vi "Teleop.vi"(10 "Match Info":T1={"Autonomous Elapsed Seconds"=0.0, "TeleOp Elapsed Seconds"=0.0, "Disabled Elapsed Seconds"=0.0, "Visited Autonomous"=FALSE, "Visited TeleOp"=FALSE, "Visited Disabled"=FALSE, "Autonomous Settings"={"Autonomous Style"=enum."Independent", "VI Refnum"=refnum}}, 11 "Call Context":T2) -> ()   [LabVIEW 2020]
doc: "This VI is called for each TeleOp packet received from the DS where the robot is not disabled. It is often used to read from the joysticks and update I/O or to update setpoints for timed control loops. It should complete and return within 20 milliseconds or it may miss DS packets."
uses:
  <vilib>/Rock Robotics/WPI/DriverStation/WPI_DriverStationDerivedRobotMode.ctl
  <vilib>/Rock Robotics/WPI/DriverStation/WPI_DriverStationMatch Info.ctl
  <vilib>/Rock Robotics/WPI/Utilities/WPI_GetSetVariantRefNum.vi
  <vilib>/Rock Robotics/Network Tables/NT Write Boolean Array.vi
  <vilib>/Rock Robotics/Network Tables/NT Write Numeric Array.vi
  Subsystems/Climber/climber_globals.vi
  Subsystems/Shooter/shooter_globals.vi
  Subsystems/Magazine/magazine_globals.vi
  Subsystems/Swerve/swerve_globals.vi
  TitanLib/Lib/TitanLib.lvlib
panel:
  out "Loop Time (ms)":u32(graph)
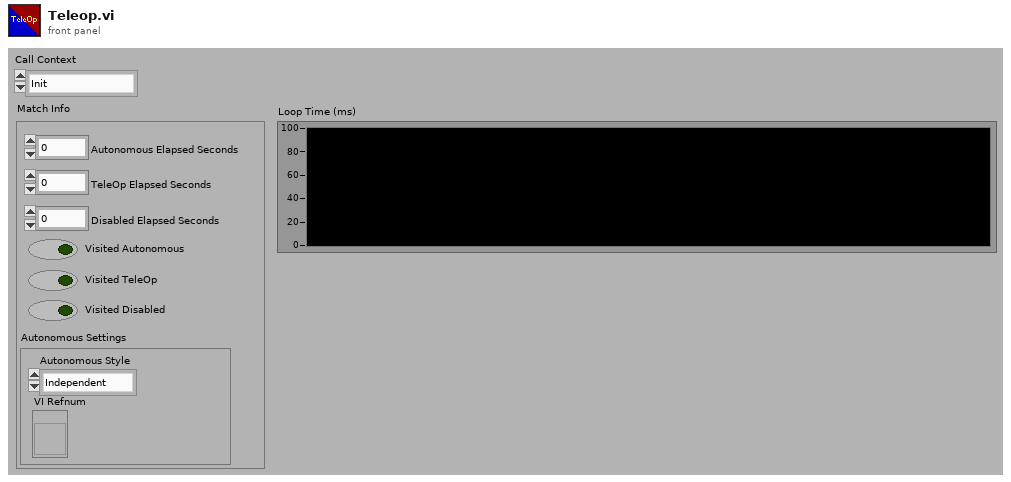
[diagram p1: front panel]
types:
  T1 = typedef "WPI_DriverStationMatch Info.ctl" = cluster{"Autonomous Elapsed Seconds":dbl, "TeleOp Elapsed Seconds":dbl, "Disabled Elapsed Seconds":dbl, "Visited Autonomous":bool, "Visited TeleOp":bool, "Visited Disabled":bool, "Autonomous Settings":cluster{"Autonomous Style":enum16{"Iterative", "Independent"}, "VI Refnum":refnum<vi>}}
  T2 = typedef "WPI_DriverStationDerivedRobotMode.ctl" = enum16{"Init", "Execute", "Stop"}
  T3 = cluster{"Left Stick X":dbl, "Left Stick Y":dbl, "Left Trigger":bool, "Right Trigger":bool, "Right Stick X":dbl, "Right Stick Y":dbl, "A":bool, "B":bool, "X":bool, "Y":bool, "Left Bumper":bool, "Right Bumper":bool, "Start":bool, "Select":bool, "Left Stick":bool, "Right Stick":bool, "POV Angle":i16, "POV Active?":bool}
  T4 = typedef "WPI_JoystickDevRef.ctl" = cluster{"Device":T5}
  T5 = typedef "WPI_JoystickDeviceEnum.ctl" = enum16{"USB 0", "USB 1", "USB 2", "USB 3", "USB 4", "USB 5"}
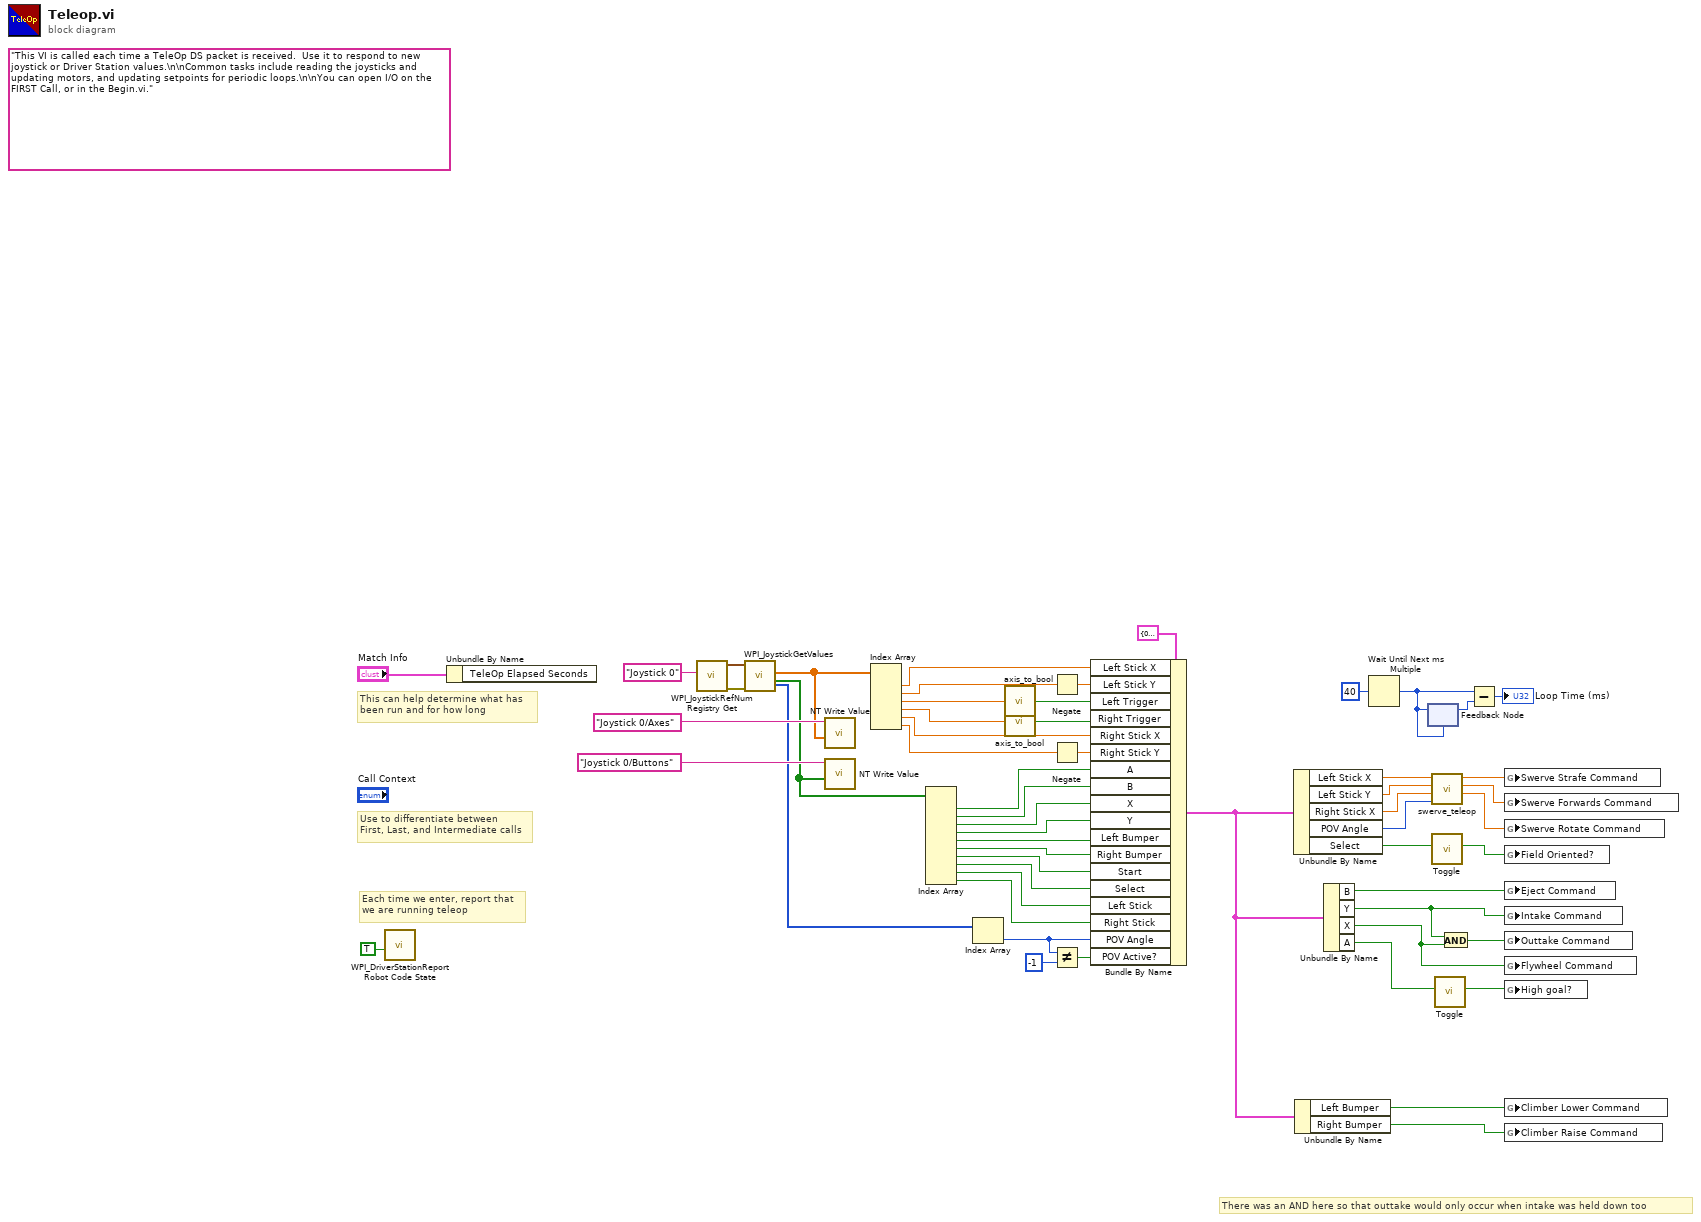
[diagram p0: block diagram]
diagram:
  (unwired) "This VI is called each time a TeleOp DS packet is received.  Use it to respond to new joystick or Driver Station values.\n\nCommon tasks include reading the joysticks and updating motors, and updating setpoints for periodic loops.\n\nYou can open I/O on the FIRST Call, or in the Begin.vi."
  # "There was an AND here so that outtake would only occur when intake was held down too"
  # "Each time we enter, report that\nwe are running teleop"
  # "Use to differentiate between\nFirst, Last, and Intermediate calls"
  # "This can help determine what has\nbeen run and for how long"
  n1 = call <vilib>:"WPI_DriverStationReport Robot Code State.vi"("TeleOp"=TRUE ("Autonomous")) -> ()  [unwired: 10 in, 1 out]
  n2 = Unbundle By Name("Match Info") -> ()  [unwired: 1 out]
  n3 = call <vilib>:"WPI_JoystickRefNum Registry Get.vi"("refnum name"="Joystick 0") -> ("error out"=w49:errorcluster, "JoystickDevRef"=w54:T4)  [unwired: 1 in, 8 out]
  n4 = call <vilib>:"WPI_JoystickGetValues.vi"("error in (no error)"=w49, "JoystickDevRef"=w54) -> ("Buttons"=w39:bool[], "Axes"=w50:dbl[], "POVs"=w28:i16[])  [unwired: 5 in, 2 out]
  n5 = call-poly <vilib>:"NT Write Value.vi"("Numeric Array"=w50, "Name"="Joystick 0/Axes") -> ()  [unwired: 9 in, 1 out]
  n6 = call-poly <vilib>:"NT Write Value.vi"("Boolean Array"=w39, "Name"="Joystick 0/Buttons") -> ()  [unwired: 9 in, 1 out]
  n7 = Index Array(array=w50) -> (element #1=w44:dbl, element #2=w43:dbl, element #3=w19:dbl, element #4=w20:dbl, element #5=w42:dbl, element #6=w41:dbl)  [unwired: 6 in]
  n8 = Index Array(array=w39) -> (element #1=w38:bool, element #2=w37:bool, element #3=w36:bool, element #4=w35:bool, element #5=w34:bool, element #6=w33:bool, element #7=w32:bool, element #8=w31:bool, element #9=w30:bool, element #10=w29:bool)  [unwired: 10 in]
  n9 = Index Array(array=w28) -> (element=w15:i16)  [unwired: 1 in]
  n10 = call "axis_to_bool.vi"("in"=w19) -> ("out"=w18:bool)
  n11 = call "axis_to_bool.vi"("in"=w20) -> ("out"=w17:bool)
  n12 = Negate(x=w43) -> (-x=w27:dbl)
  n13 = Negate(x=w41) -> (-x=w26:dbl)
  n14 = Not Equal?(x=w15, y=i16 -1) -> (x != y?=w16:bool)
  n15 = Bundle By Name(cluster=T3 {"Left Stick X"=0.0, "Left Stick Y"=0.0, "Left Trigger"=FALSE, "Right Trigger"=FALSE, "Right Stick X"=0.0, "Right Stick Y"=0.0, "A"=FALSE, "B"=FALSE, "X"=FALSE, "Y"=FALSE, "Left Bumper"=FALSE, "Right Bumper"=FALSE, "Start"=FALSE, "Select"=FALSE, "Left Stick"=FALSE, "Right Stick"=FALSE, "POV Angle"=0, "POV Active?"=FALSE} ("input cluster"), "Left Stick X"=w44, "Left Stick Y"=w27, "Left Trigger"=w18, "Right Trigger"=w17, "Right Stick X"=w42, "Right Stick Y"=w26, "A"=w38, "B"=w37, "X"=w36, "Y"=w35, "Left Bumper"=w34, "Right Bumper"=w33, "Start"=w32, "Select"=w31, "Left Stick"=w30, "Right Stick"=w29, "POV Angle"=w15, "POV Active?"=w16) -> (w21:T3)
  n16 = Unbundle By Name(w21) -> ("Left Stick X"=w25:dbl, "Left Stick Y"=w24:dbl, "Right Stick X"=w23:dbl, "POV Angle"=w22:i16, "Select"=w10:bool)
  n17 = Unbundle By Name(w21) -> ("Left Bumper"=w12:bool, "Right Bumper"=w11:bool)
  n18 = Unbundle By Name(w21) -> ("B"=w13:bool, "Y"=w5:bool, "X"=w4:bool, "A"=w2:bool)
  n19 = Wait Until Next ms Multiple(millisecond multiple=u32 40) -> (millisecond timer value=w46:u32)
  n20 = feedback #1(w46) -> (w48:u32)
  n21 = feedback-in #1(w46) -> ()
  n22 = call "swerve_teleop.vi"("POV Angle"=w22, "Rotate Axis"=w23, "Forwards Axis"=w24, "Strafe Axis"=w25) -> ("Rotate Command"=w9:dbl, "Forwards Command"=w7:dbl, "Strafe Command"=w8:dbl)  [unwired: 5 in]
  n23 = call "Toggle.vi"("Input"=w10) -> ("Output"=w6:bool)  [unwired: 10 in]
  n24 = call "Toggle.vi"("Input"=w2) -> ("Output"=w1:bool)  [unwired: 10 in]
  n25 = And(x=w5, y=w4) -> (x .and. y?=w3:bool)
  n26 = Subtract(x=w46, y=w48) -> (x-y=→"Loop Time (ms)":u32)
  n27 = global write "swerve_globals.vi" "Swerve Strafe Command"(w8) -> ()
  n28 = global write "swerve_globals.vi" "Swerve Forwards Command"(w7) -> ()
  n29 = global write "swerve_globals.vi" "Swerve Rotate Command"(w9) -> ()
  n30 = global write "swerve_globals.vi" "Field Oriented?"(w6) -> ()
  n31 = global write "magazine_globals.vi" "Eject Command"(w13) -> ()
  n32 = global write "magazine_globals.vi" "Intake Command"(w5) -> ()
  n33 = global write "magazine_globals.vi" "Outtake Command"(w3) -> ()
  n34 = global write "shooter_globals.vi" "Flywheel Command"(w4) -> ()
  n35 = global write "shooter_globals.vi" "High goal?"(w1) -> ()
  n36 = global write "climber_globals.vi" "Climber Lower Command"(w12) -> ()
  n37 = global write "climber_globals.vi" "Climber Raise Command"(w11) -> ()
